vi "Get Waveform.vi"(6 "timeout (ms)":i32=5000, 8 "error in":errorcluster, 11 "gRPC ID":T3) -> (0 "error out":errorcluster, 2 "Waveforms":T1, 3 "gRPC ID out":T3)   [LabVIEW 2021, in "CIFWaveformMonitorWrapper.lvlib"]
uses:
  CIFWaveformMonitorWrapper.lvlib
  <vilib>/gRPC/LabVIEW gRPC Library/Shared/grpcId.ctl
  CIFWaveformMonitor_client/CIFWaveformMonitor_client.lvlib
  <vilib>/gRPC/LabVIEW gRPC Library/grpc-lvsupport-release.lvlib
  CIFWaveformMonitor_client/RPC Messages/cif_waveformmonitor_Waveform.ctl
  CIFWaveformMonitor_client/RPC Messages/cif_waveformmonitor_Waveforms.ctl
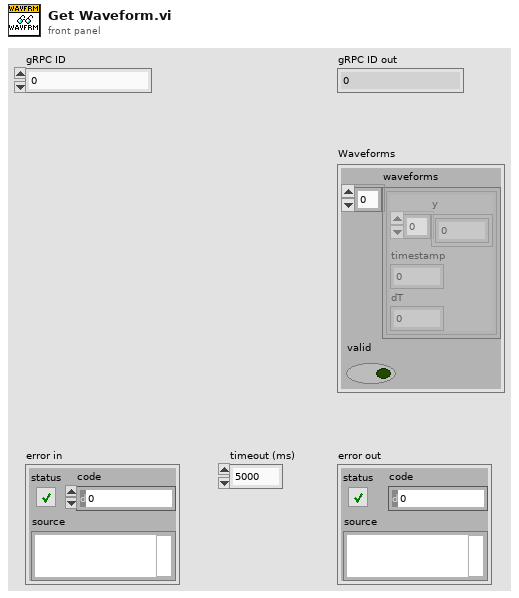
[diagram p1: front panel]
types:
  T1 = typedef "CIFWaveformMonitor_client.lvlib/cif_waveformmonitor_Waveforms.ctl" = cluster{"waveforms":T2[], "valid":bool}
  T2 = typedef "CIFWaveformMonitor_client.lvlib/cif_waveformmonitor_Waveform.ctl" = cluster{"y":dbl[], "timestamp":u64, "dT":dbl}
  T3 = typedef "grpc-lvsupport-release.lvlib/grpcId.ctl" = u64
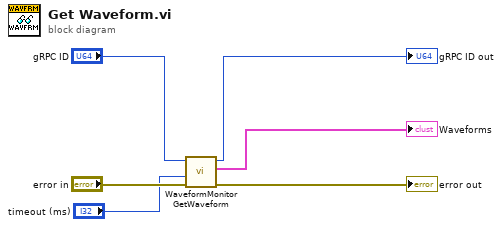
[diagram p0: block diagram]
diagram:
  n1 = call "WaveformMonitor GetWaveform.vi"("error in"="error in", "timeout (ms)"="timeout (ms)", "gRPC ID"="gRPC ID") -> ("error out"=→"error out":errorcluster, "Response Data"=→"Waveforms":T1, "gRPC ID out"=→"gRPC ID out":T3)  [unwired: 6 in]
